vi "absorptionImaging.vi"() -> ()   [LabVIEW 2011, in "run.lvlib"]
uses:
  testing/run.lvlib
  Tools/Filing/FileNeologist/FileNeologist.lvclass
panel:
  out "Image":T1(plugin-control)
  in  "Save":bool=TRUE
  out "Images Taken":i32
  out "path":path
  in  "number of images":i32=4
  out "Board Parameters":T2 {"Vertical bin" items=["1", "2"]; "Horizontal bin" items=["1", "2"]}
  in  "gain":i32(ring) items=["Low (X1)", "High (X2)"]
  in  "exp time":i32(slide)=90 min=1 max=10000 scale=0.0..300.0
  in  "V bin":i32(ring) items=["1", "2"]
  in  "H bin":i32(ring) items=["1", "2"]
  in  "trigger":bool=TRUE
  in  "Exposure mode":u16(ring)=1 items=["Asynch shutter", "Double shot", "Video mode", "Auto exposure"]
  out "ccdtemp":i32(slide) scale=0.0..100.0
  in  "stop":bool
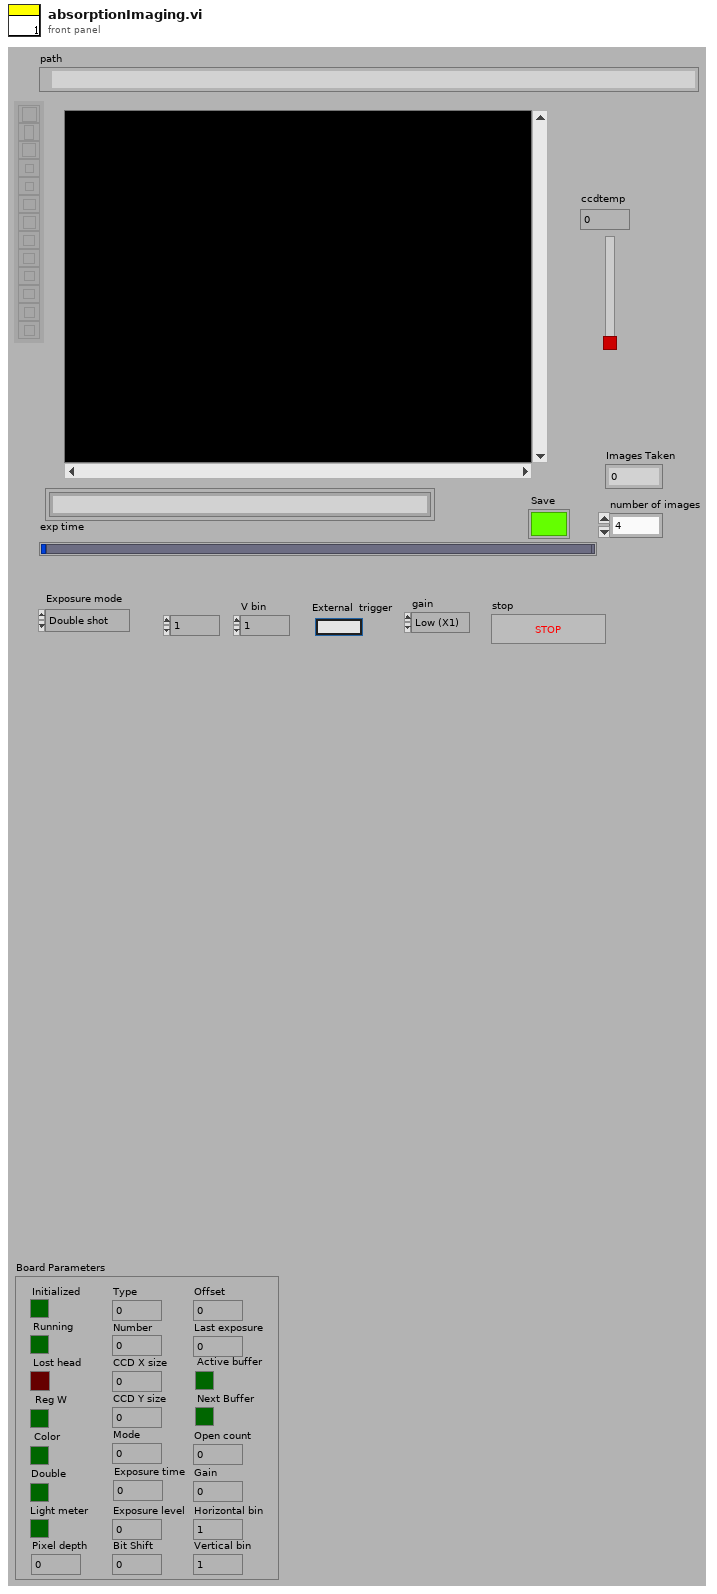
[diagram p1: front panel]
types:
  T1 = typedef "IMAQ Image.ctl" = refnum<image>
  T2 = cluster{"Type":u32, "Number":u32, "Initialized":bool, "Running":bool, "Lost head":bool, "CCD X size":u32, "CCD Y size":u32, "Mode":u32, "Exposure time":u32, "Exposure level":u32, "Horizontal bin":u32, "Vertical bin":u32, "Reg W":bool, "Gain":u32, "Pixel depth":i32, "Bit Shift":u32, "Offset":u32, "Last exposure":u32, "Double ":bool, "Light meter":bool, "Color":bool, "Open count":u32, "Active buffer":bool, "Next Buffer":bool}
  T3 = typedef "Image Type" = u32
  T4 = cluster{"ccdxsize":i32, "ccdy":i32, "pictx":i32, "picty":i32, "bitspixel":i32}
  T5 = cluster{"Write":bool, "Write done":bool, "Queued":bool, "Cancelled":bool, "Select":bool, "Select done":bool, "Burst":bool, "Size":bool, "Event":bool, "Timeout":bool, "Open":i32, "Map":i32, "Exposure":i32[], "Offset":i32[], "Size":i32[], "Transfer":i32[], "Total Size":i32}
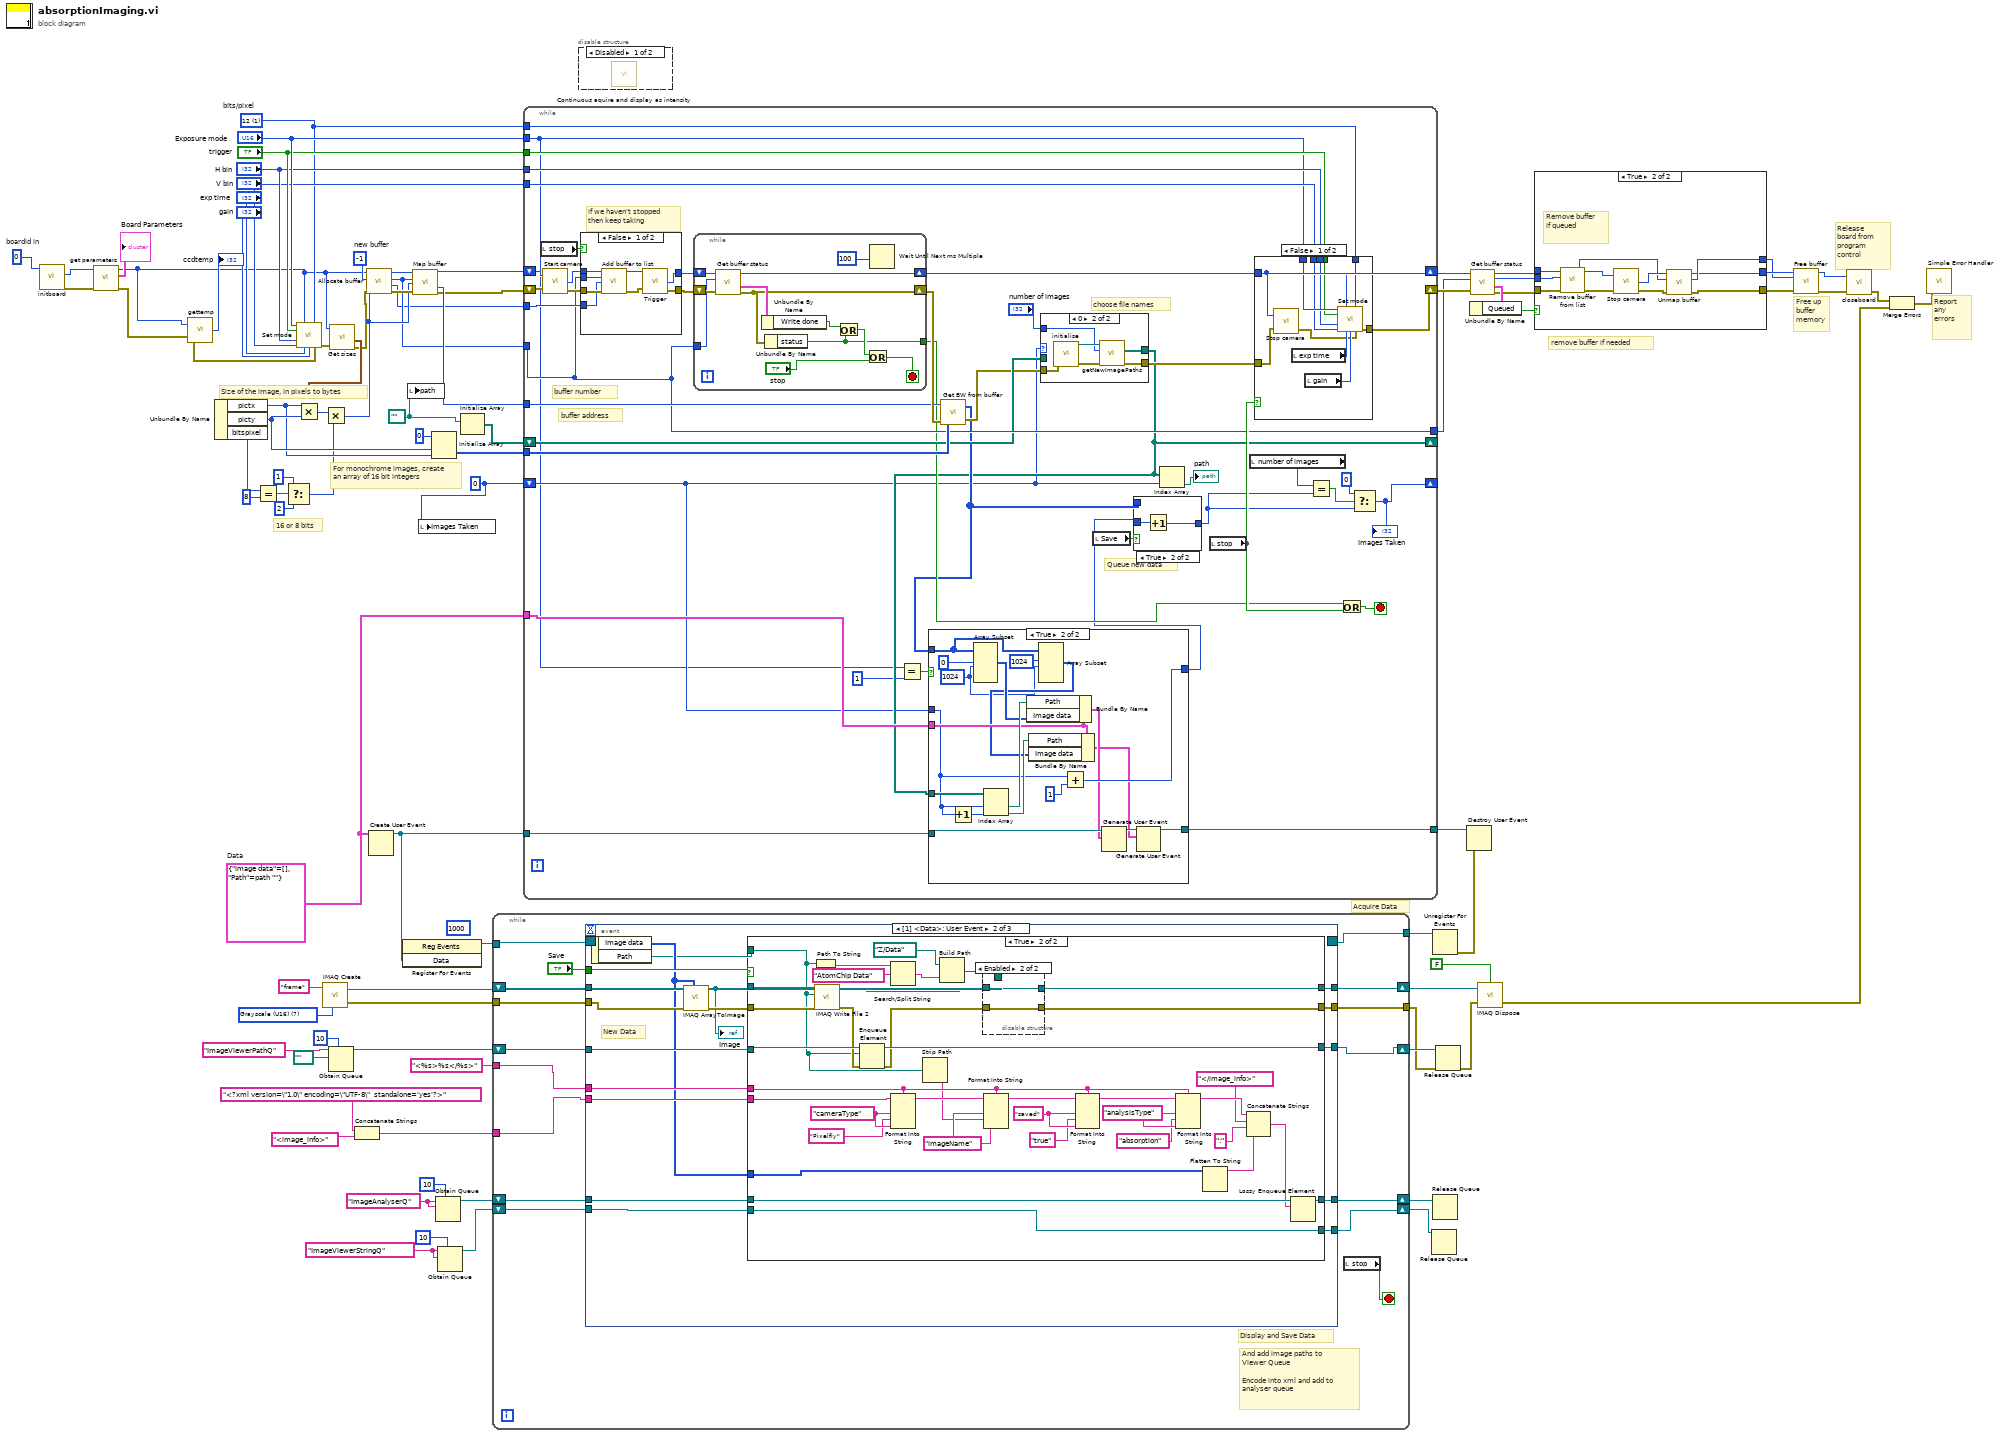
[diagram p0: block diagram]
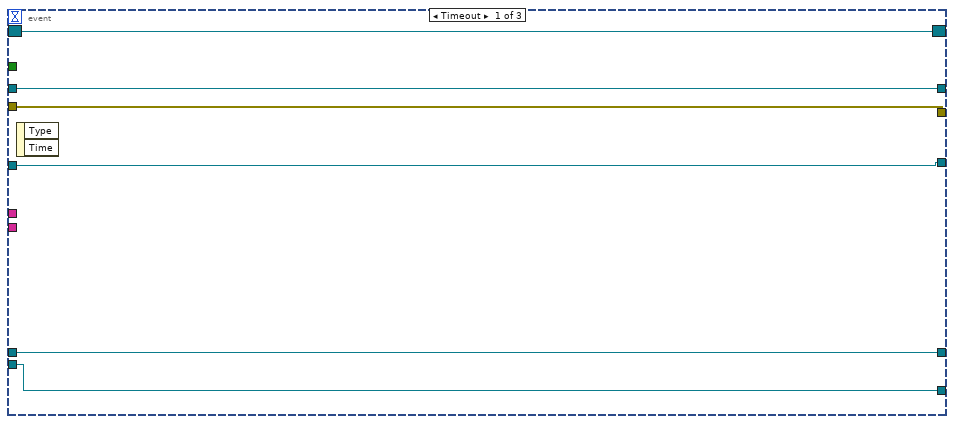
[diagram p2: hidden frame]
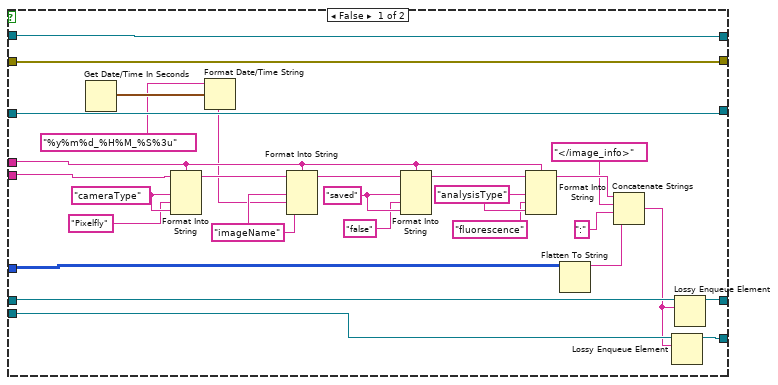
[diagram p3: hidden frame]
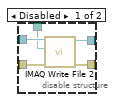
[diagram p4: hidden frame]
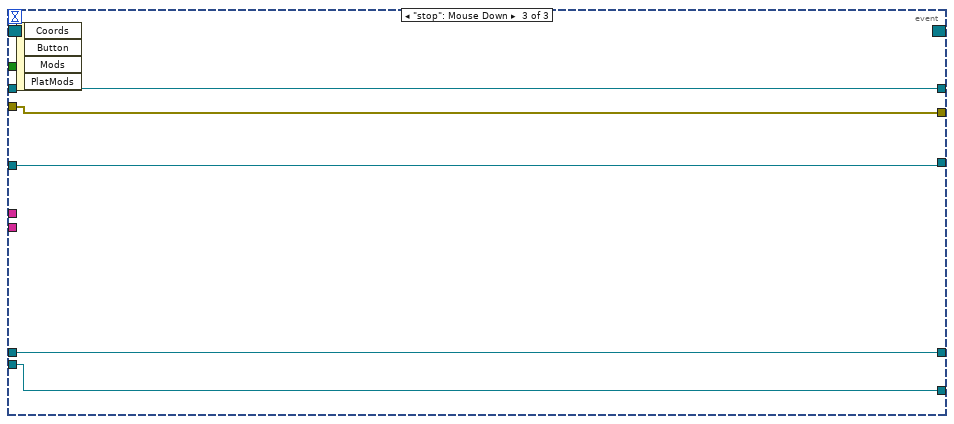
[diagram p5: hidden frame]
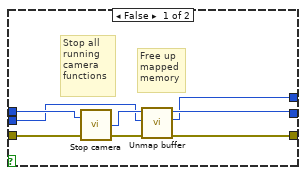
[diagram p7: hidden frame]
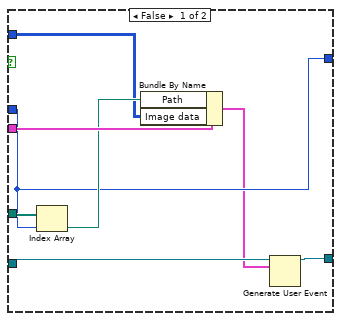
[diagram p8: hidden frame]
diagram:
  (unwired) 1000
  w16 = "ImageViewerStringQ"
  w20 = "ImageAnalyserQ"
  w5 = cluster{"Image data":u16[][], "Path":path} {"Image data"=[], "Path"=path ""}  # Data
  w35 = T3 7 items=["Grayscale (U8)", "Grayscale (I16)", "Grayscale (SGL)", "Complex (CSG)", "RGB (U32)", "HSL (U32)", "RGB (U64)", "Grayscale (U16)"] ("Image Type")
  w31 = path ""
  w30 = 0
  w54 = 1 items=["8", "12"]  # bits/pixel
  w70 = -1  # new buffer
  w74 = 0  # boardid in
  # "Acquire Data"
  # "remove buffer if needed"
  # "Report any errors"
  # "Release board from program control"
  # "Free up buffer memory"
  # "16 or 8 bits"
  # "For monochrome images, create an array of 16 bit integers"
  # "Size of the image, in pixels to bytes"
  n1 = call <instrlib>:"initboard.vi"("boardid in"=w74) -> ("boardid"=w86:i32, "error out"=w44:errorcluster)  [unwired: 3 in, 1 out]
  n2 = call <instrlib>:"get parameters.vi"("error in (no error)"=w44, "Handle in"=w86) -> ("error out"=w10:errorcluster, "Board Parameters"=→"Board Parameters":T2, "Error out"=w7:i32)  [unwired: 2 in, 1 out]
  n3 = call <instrlib>:"gettemp.vi"("Handle in"=w7, "error in (no error)"=w10) -> ("ccdtemp"=→"ccdtemp":i32, "error out"=w87:errorcluster)  [unwired: 1 out]
  n4 = call <instrlib>:"Set mode.vi"("Exposure mode"="Exposure mode", "Handle in"=w7, "bits/pixel"=w54, "trigger"="trigger", "H bin"="H bin", "V bin"="V bin", "exp time"="exp time", "gain"="gain", "error in (no error)"=w87) -> ("error out"=w9:errorcluster)  [unwired: 6 in]
  n5 = call "IMAQ Create"("Image Name"="frame", "Image Type"=w35) -> ("New Image"=w34:T1, "error out"=w33:errorcluster)  [unwired: 3 in]
  n6 = Obtain Queue(max queue size (-1, unlimited)=10, name (unnamed)="ImageViewerPathQ", element data type=path "") -> (queue out=w28:refnum<queue>)  [unwired: 2 in, 2 out]
  n7 = call <instrlib>:"Get sizes.vi"("Handle in"=w7, "error in (no error)"=w9) -> ("Picture parameters"=w82:T4, "error out"=w8:errorcluster)  [unwired: 1 in, 2 out]
  n8 = Unbundle By Name(w82) -> ("pictx"=w79:i32, "picty"=w80:i32, "bitspixel"=w81:i32)
  n9 = Equal?(x=w81, y=8) -> (x = y?=w78:bool)
  n10 = Select(t=1, s=w78, f=2) -> (s? t:f=w75:i32)
  n11 = Multiply(x=w79, y=w80) -> (x*y=w38:i32)
  n12 = Multiply(x=w38, y=w75) -> (x*y=w72:i32)
  n13 = Concatenate Strings("<?xml version=\"1.0\" encoding=\"UTF-8\"  standalone='yes'?>", "<image_info>") -> (w22:string)
  n14 = call <instrlib>:"Allocate buffer.vi"("error in (no error)"=w8, "Size request"=w72, "Buffer request"=w70, "Handle in"=w7) -> ("error out"=w85:errorcluster, "Size"=w52:i32, "Buffer number"=w53:i32, "Handle out"=w88:i32)
  n15 = Create User Event(user event datatype=w5) -> (user event=w3:refnum<user-event>)  [unwired: 1 in, 1 out]
  n16 = register-events(w3) -> (reference out=w4:refnum<event-registration>)  [unwired: 2 in, 1 out]
  n17 = local write "path"(w31) -> ()
  n18 = call <instrlib>:"Map buffer.vi"("Handle in"=w88, "Buffer in"=w53, "size"=w72, "error in (no error)"=w85) -> ("Handle out"=w51:i32, "Buffer address"=w73:i32, "error out"=w50:errorcluster)  [unwired: 8 in, 1 out]
  n19 = local write "Images Taken"(w30) -> ()
  n20 = Initialize Array(u16 0 ("16 bit integers"), w80, w79) -> (w71:u16[][])
  n21 = Obtain Queue(max queue size (-1, unlimited)=10, name (unnamed)=w20, element data type=w20) -> (queue out=w19:refnum<queue>)  [unwired: 2 in, 2 out]
  n22 = Obtain Queue(max queue size (-1, unlimited)=10, name (unnamed)=w16, element data type=w16) -> (queue out=w17:refnum<queue>)  [unwired: 2 in, 2 out]
  n23 = Initialize Array(w31) -> (w37:path[])  [unwired: 1 in]
  n24 = while {
    tunnel: w33 -> [w103]
    tunnel: [w99] -> w26
    shift-right: [w101] -> w27
    shift-left: w28 -> [w102]
    shift-right: [w100] -> w32
    shift-left: w34 -> [w104]
    tunnel: w22 -> [w94]
    tunnel: "<%s>%s</%s>" -> [w93]
    shift-right: [w98] -> w18
    shift-left: w19 -> [w96]
    shift-right: [w97] -> w15
    shift-left: w17 -> [w95]
    tunnel: w4 -> [w91]
    tunnel: [w90] -> w2
    stop <- w89 stop-if-true
    # "Display and Save Data"
    # "And add image paths to \nViewer Queue\n\nEncode into xml and add to\nanalyser queue"
    n25 = event shown="[1] <Data>: User Event" {
      selector: w91 -> [w105 _ _]
      dyn-events: [w105 _ _] -> w90
      timeout: _ -> [_ _ _]
      tunnel: w104 -> [w110 w126 w202]
      tunnel: w103 -> [w109 w125 w201]
      tunnel: w102 -> [w108 w124 w200]
      tunnel: [w108 w123 w200] -> w101
      tunnel: [w110 w122 w202] -> w100
      tunnel: [w109 w121 w201] -> w99
      tunnel: [w107 w120 w204] -> w98
      tunnel: [w106 w119 w203] -> w97
      tunnel: w96 -> [w107 w118 w204]
      tunnel: w95 -> [w106 w117 w203]
      tunnel: w94 -> [_ w116 _]
      tunnel: w93 -> [_ w115 _]
      tunnel: "Save" -> [_ w114 _]
      event Timeout {
        n26 = event-data() -> ()  [unwired: 1 in, 2 out]
      }
      event User Event {
        # "New Data"
        n27 = event-data() -> ("Image data"=w112:u16[][], "Path"=w111:path)  [unwired: 1 in]
        n28 = call "IMAQ ArrayToImage"("Image Pixels (U16)"=w112, "error in (no error)"=w125, "Image"=w126) -> ("error out"=w127:errorcluster, "Image Out"=w113:T1)  [unwired: 7 in]
        "Image" <- w113
        n29 = case shown="True" w114 {
          tunnel: [w155 w159] -> w122
          tunnel: [w154 w157] -> w121
          tunnel: w127 -> [w154 w192]
          tunnel: w113 -> [w155 w191]
          tunnel: w111 -> [_ w165]
          tunnel: w124 -> [w153 w190]
          tunnel: [w153 w188] -> w123
          tunnel: w115 -> [w137 w177]
          tunnel: w116 -> [w136 w176]
          tunnel: w112 -> [w135 w171]
          tunnel: w118 -> [w152 w169]
          tunnel: [w129 w167] -> w120
          tunnel: w117 -> [w131 w166]
          tunnel: [w130 w166] -> w119
          frame False {
            w149 = "analysisType"
            w147 = "saved"
            w143 = "imageName" ("Key")
            w142 = "cameraType"
            n30 = Get Date/Time In Seconds() -> (seconds since 1Jan1904=w134:timestamp)
            n31 = Format Into String(format string=w137, initial string=w136, w142, "Pixelfly", w142) -> (resulting string=w145:string)  [unwired: 1 in, 1 out]
            n32 = Format Date/Time String(time format string (%c)="%y%m%d_%H%M_%S%3u", seconds (now)=w134) -> (date/time string=w132:string)  [unwired: 1 in]
            n33 = Format Into String(format string=w137, initial string=w145, w143, w132, w143) -> (resulting string=w146:string)  [unwired: 1 in, 1 out]
            n34 = Format Into String(format string=w137, initial string=w146, w147, "false", w147) -> (resulting string=w150:string)  [unwired: 1 in, 1 out]
            n35 = Format Into String(format string=w137, initial string=w150, w149, "fluorescence", w149) -> (resulting string=w151:string)  [unwired: 1 in, 1 out]
            n36 = Flatten To String(anything=w135) -> (data string=w138:string)  [unwired: 3 in, 2 out]
            n37 = Concatenate Strings(w151, "</image_info>", ":", w138) -> (w128:string)
            n38 = Lossy Enqueue Element(queue=w131, element=w128) -> (queue out=w130:refnum<queue>)  [unwired: 1 in, 3 out]
            n39 = Lossy Enqueue Element(queue=w152, element=w128) -> (queue out=w129:refnum<queue>)  [unwired: 1 in, 3 out]
          }
          frame True {
            w185 = "analysisType"
            w183 = "saved"
            w179 = "imageName" ("Key")
            w178 = "cameraType"
            n40 = Path To String(path=w165) -> (string=w164:string)
            n41 = call-poly "IMAQ Write File 2"("error in (no error)"=w192, "File Path"=w165, "Image"=w191) -> ("error out"=w189:errorcluster, "Image Out (duplicate)"=w160:T1)  [unwired: 7 in]
            n42 = Enqueue Element(queue=w190, element=w165, error in (no error)=w189) -> (queue out=w188:refnum<queue>, error out=w158:errorcluster)  [unwired: 1 in, 1 out]
            n43 = Search/Split String(string=w164, search string/char (-)="AtomChip Data") -> (match + rest of string=w162:string)  [unwired: 1 in, 2 out]
            n44 = Format Into String(format string=w177, initial string=w176, w178, "Pixelfly", w178) -> (resulting string=w181:string)  [unwired: 1 in, 1 out]
            n45 = Strip Path(path=w165) -> (name=w175:string)  [unwired: 1 out]
            n46 = Build Path(base path=path "Z:/Data", name or relative path=w162) -> (appended path=w156:path)
            n47 = disable-structure shown="Enabled" {
              disable-tunnel: w160 -> [w197 w199]
              disable-tunnel: [w196 w199] -> w159
              disable-tunnel: w158 -> [w195 w198]
              disable-tunnel: [w194 w198] -> w157
              disable-tunnel: w156 -> [w193 _]
              frame Disabled {
                n48 = call-poly "IMAQ Write File 2"("error in (no error)"=w195, "File Path"=w193, "Image"=w197) -> ("error out"=w194:errorcluster, "Image Out (duplicate)"=w196:T1)  [unwired: 7 in]
              }
              frame Enabled {
              }
            }
            n49 = Format Into String(format string=w177, initial string=w181, w179, w175, w179) -> (resulting string=w182:string)  [unwired: 1 in, 1 out]
            n50 = Format Into String(format string=w177, initial string=w182, w183, "true", w183) -> (resulting string=w186:string)  [unwired: 1 in, 1 out]
            n51 = Format Into String(format string=w177, initial string=w186, w185, "absorption", w185) -> (resulting string=w187:string)  [unwired: 1 in, 1 out]
            n52 = Flatten To String(anything=w171) -> (data string=w170:string)  [unwired: 3 in, 2 out]
            n53 = Concatenate Strings(w187, "</image_info>", ":", w170) -> (w168:string)
            n54 = Lossy Enqueue Element(queue=w169, element=w168) -> (queue out=w167:refnum<queue>)  [unwired: 1 in, 3 out]
          }
        }
      }
      event "stop": Mouse Down {
        n55 = event-data() -> ()  [unwired: 1 in, 4 out]
      }
    }
    n56 = local read "stop"() -> (w89:bool)
  }
  n57 = while {
    tunnel: w53 -> [w228]
    shift-right: [w233] -> w65
    shift-left: w51 -> [w232]
    shift-right: [w234] -> w64
    shift-left: w50 -> [w227]
    tunnel: w73 -> [w242]
    tunnel: w71 -> [w241]
    tunnel: "Exposure mode" -> [w207]
    tunnel: "trigger" -> [w237]
    tunnel: "H bin" -> [w236]
    tunnel: "V bin" -> [w235]
    tunnel: w54 -> [w238]
    tunnel: w52 -> [w240]
    tunnel: [w228] -> w48
    shift-right: [w226] -> _
    shift-left: w30 -> [w208]
    shift-right: [w212] -> _
    shift-left: w37 -> [w222]
    tunnel: w5 -> [w213]
    tunnel: w3 -> [w206]
    tunnel: [w205] -> w6
    stop <- w239 stop-if-true
    # "Queue new data"
    # "choose file names"
    # "buffer address"
    # "buffer number"
    # "if we haven't stopped\nthen keep taking"
    n58 = local read "stop"() -> (w246:bool)
    n59 = call <instrlib>:"Start camera.vi"("Handle in"=w232, "error in (no error)"=w227) -> ("Handle out"=w231:i32, "error out"=w230:errorcluster)  [unwired: 1 out]
    n60 = case shown="False" w246 {
      tunnel: w230 -> [w303 w304]
      tunnel: [w301 w304] -> w245
      tunnel: w231 -> [w300 w305]
      tunnel: [w298 w305] -> w244
      tunnel: w228 -> [w297 _]
      tunnel: w240 -> [w296 _]
      frame False {
        n61 = call <instrlib>:"Add buffer to list.vi"("Handle in"=w300, "Buffer in"=w297, "size"=w296, "error in (no error)"=w303) -> ("Handle out"=w299:i32, "error out"=w302:errorcluster)  [unwired: 9 in, 1 out]
        n62 = call <instrlib>:"Trigger.vi"("Handle in"=w299, "error in (no error)"=w302) -> ("Handle out"=w298:i32, "error out"=w301:errorcluster)  [unwired: 1 out]
      }
      frame True {
      }
    }
    n63 = while {
      tunnel: w228 -> [w310]
      shift-right: [w308] -> w233
      shift-left: w244 -> [w311]
      shift-right: [w309] -> w243
      shift-left: w245 -> [w312]
      tunnel: [w307] -> w216
      stop <- w313 stop-if-true
      n64 = call <instrlib>:"Get buffer status.vi"("error in (no error)"=w312, "Buffer request"=w310, "Handle in"=w311) -> ("error out"=w309:errorcluster, "Buffer status"=w317:T5, "Handle out"=w308:i32)  [unwired: 1 in, 1 out]
      n65 = Unbundle By Name(w317) -> ("Write done"=w316:bool)
      n66 = Unbundle By Name(w309) -> ("status"=w307:bool)
      n67 = Or(x=w316, y=w307) -> (x .or. y?=w315:bool)
      n68 = Or(x=w315, y="stop") -> (x .or. y?=w313:bool)
      n69 = Wait Until Next ms Multiple(millisecond multiple=100) -> ()  [unwired: 1 out]
    }
    n70 = Equal?(x=w207, y=1) -> (x = y?=w211:bool)
    n71 = call <instrlib>:"Get BW from buffer.vi"("error in (no error)"=w243, "Array input"=w241, "Buffer address"=w242) -> ("error out"=w221:errorcluster, "Image data"=w215:u16[][])
    n72 = case shown="0" w208 {
      tunnel: [w275 w279] -> w212
      tunnel: w222 -> [w275 _]
      tunnel: w221 -> [w274 w278]
      tunnel: [w274 w277] -> w217
      tunnel: "number of images" -> [_ w276]
      frame Default {
      }
      frame 0 {
        n73 = call "initialise.vi"("error in (no error)"=w278) -> ("error out"=w280:errorcluster, "FileNeologist out"=w281:refnum<class "FileNeologist.lvclass">)  [unwired: 9 in]
        n74 = call "getNewImagePaths.vi"("error in (no error)"=w280, "numberOfImages"=w276, "FileNeologist in"=w281) -> ("error out"=w277:errorcluster, "Paths"=w279:path[])  [unwired: 6 in, 1 out]
      }
    }
    n75 = case shown="True" w211 {
      tunnel: w213 -> [w254 w266]
      tunnel: w215 -> [w251 w272]
      tunnel: w212 -> [w253 w270]
      tunnel: w208 -> [w250 w263]
      tunnel: [w250 w261] -> w209
      tunnel: w206 -> [w248 w259]
      tunnel: [w249 w255] -> w205
      frame False {
        n76 = Index Array(array=w253, index=w250) -> (element=w252:path)
        n77 = Bundle By Name(cluster=w254, "Path"=w252, "Image data"=w251) -> (w247:cluster{"Image data":u16[][], "Path":path})
        n78 = Generate User Event(user event=w248, event data cluster=w247) -> (user event out=w249:refnum<user-event>)  [unwired: 1 in, 1 out]
      }
      frame True {
        w260 = 1024
        n79 = Increment(x=w263) -> (x+1=w269:i32)
        n80 = Array Subset(array=w272, index (row)=0, length (row)=w260) -> (w267:u16[][])  [unwired: 2 in]
        n81 = Index Array(array=w270, index #1=w263, index #2=w269) -> (element #1=w268:path, element #2=w265:path)
        n82 = Bundle By Name(cluster=w266, "Path"=w268, "Image data"=w267) -> (w258:cluster{"Image data":u16[][], "Path":path})
        n83 = Array Subset(array=w272, index (row)=1024, length (row)=w260) -> (w264:u16[][])  [unwired: 2 in]
        n84 = Bundle By Name(cluster=w266, "Path"=w265, "Image data"=w264) -> (w256:cluster{"Image data":u16[][], "Path":path})
        n85 = Add(x=w263, y=1) -> (x+y=w261:i32)
        n86 = Generate User Event(user event=w259, event data cluster=w258) -> (user event out=w257:refnum<user-event>)  [unwired: 1 in, 1 out]
        n87 = Generate User Event(user event=w257, event data cluster=w256) -> (user event out=w255:refnum<user-event>)  [unwired: 1 in, 1 out]
      }
    }
    n88 = local read "Save"() -> (w218:bool)
    n89 = case shown="True" w218 {
      tunnel: w209 -> [_ w283]
      tunnel: [_ w282] -> w224
      tunnel: w215 -> [_ _]
      frame False {
      }
      frame True {
        n90 = Increment(x=w283) -> (x+1=w282:i32)
      }
    }
    n91 = Index Array(array=w212, index=w208) -> (element=→"path":path)
    n92 = local read "stop"() -> (w229:bool)
    n93 = local read "number of images"() -> (w219:i32)
    n94 = case shown="False" w229 {
      tunnel: w238 -> [w294 _]
      tunnel: w207 -> [w293 _]
      tunnel: w237 -> [w292 _]
      tunnel: w236 -> [w291 _]
      tunnel: w235 -> [w290 _]
      tunnel: [w287 w295] -> w234
      tunnel: w233 -> [w285 _]
      tunnel: w217 -> [w284 w295]
      frame False {
        n95 = call <instrlib>:"Stop camera.vi"("Handle in"=w285, "error in (no error)"=w284) -> ("error out"=w286:errorcluster)  [unwired: 2 out]
        n96 = local read "exp time"() -> (w289:i32)
        n97 = local read "gain"() -> (w288:i32)
        n98 = call <instrlib>:"Set mode.vi"("Exposure mode"=w293, "Handle in"=w285, "bits/pixel"=w294, "trigger"=w292, "H bin"=w291, "V bin"=w290, "exp time"=w289, "gain"=w288, "error in (no error)"=w286) -> ("error out"=w287:errorcluster)  [unwired: 6 in]
      }
      frame True {
      }
    }
    n99 = Equal?(x=w219, y=w224) -> (x = y?=w225:bool)
    n100 = Or(x=w216, y=w229) -> (x .or. y?=w239:bool)
    n101 = Select(t=0, s=w225, f=w224) -> (s? t:f=w226:i32)
    "Images Taken" <- w226
  }
  n102 = disable-structure shown="Disabled" {
    frame Disabled {
      n103 = call <instrlib>:"Continuous aquire and display as intensity.vi"() -> ()  [unwired: 1 in]
    }
    frame Enabled {
    }
  }
  n104 = Release Queue(queue=w15) -> ()  [unwired: 2 in, 3 out]
  n105 = Unregister For Events(event registration refnum=w2) -> (error out=w1:errorcluster)  [unwired: 1 in]
  n106 = Release Queue(queue=w18) -> ()  [unwired: 2 in, 3 out]
  n107 = Release Queue(queue=w27, error in (no error)=w26) -> (error out=w25:errorcluster)  [unwired: 1 in, 2 out]
  n108 = Destroy User Event(user event=w6, error in=w1) -> ()  [unwired: 1 out]
  n109 = call <instrlib>:"Get buffer status.vi"("error in (no error)"=w64, "Buffer request"=w48, "Handle in"=w65) -> ("error out"=w66:errorcluster, "Buffer status"=w67:T5, "Buffer number"=w63:i32, "Handle out"=w62:i32)  [unwired: 1 in]
  n110 = Unbundle By Name(w67) -> ("Queued"=w49:bool)
  n111 = call "IMAQ Dispose"("All Images? (No)"=FALSE, "Image"=w32, "error in (no error)"=w25) -> ("error out"=w40:errorcluster)  [unwired: 3 in]
  n112 = case shown="True" w49 {
    tunnel: w66 -> [w322 w336]
    tunnel: [w320 w326] -> w45
    tunnel: w63 -> [w321 w335]
    tunnel: w62 -> [w323 w334]
    tunnel: [w319 w327] -> w47
    tunnel: [w318 w328] -> w46
    frame False {
      # "Free up mapped memory"
      # "Stop all running camera functions"
      n113 = call <instrlib>:"Stop camera.vi"("Handle in"=w323, "error in (no error)"=w322) -> ("Handle out"=w325:i32, "error out"=w324:errorcluster)  [unwired: 1 out]
      n114 = call <instrlib>:"Unmap buffer.vi"("error in (no error)"=w324, "Buffer in"=w321, "Handle in"=w325) -> ("error out"=w320:errorcluster, "Buffer number"=w318:i32, "Handle out"=w319:i32)  [unwired: 2 in]
    }
    frame True {
      # "Remove buffer if queued"
      n115 = call <instrlib>:"Remove buffer from list.vi"("error in (no error)"=w336, "Buffer in"=w335, "Handle in"=w334) -> ("error out"=w333:errorcluster, "Buffer number"=w329:i32, "Handle out"=w332:i32)  [unwired: 2 in]
      n116 = call <instrlib>:"Stop camera.vi"("Handle in"=w332, "error in (no error)"=w333) -> ("Handle out"=w330:i32, "error out"=w331:errorcluster)  [unwired: 1 out]
      n117 = call <instrlib>:"Unmap buffer.vi"("error in (no error)"=w331, "Buffer in"=w329, "Handle in"=w330) -> ("error out"=w326:errorcluster, "Buffer number"=w328:i32, "Handle out"=w327:i32)  [unwired: 2 in]
    }
  }
  n118 = call <instrlib>:"Free buffer.vi"("error in (no error)"=w45, "Buffer in"=w46, "Handle in"=w47) -> ("error out"=w68:errorcluster, "Handle out"=w61:i32)  [unwired: 2 in, 1 out]
  n119 = call <instrlib>:"closeboard.vi"("Handle in"=w61, "error in (no error)"=w68) -> ("error out"=w42:errorcluster)  [unwired: 2 out]
  n120 = Merge Errors(w42, w40) -> (w41:errorcluster)
  n121 = call <vilib>:"Simple Error Handler.vi"("error in (no error)"=w41) -> ()  [unwired: 4 in, 5 out]
